vi "平面三体问题v7.vi"() -> ()   [LabVIEW 2018]
uses:
  <vilib>/Analysis/1siggen.llb/Ramp Pattern by Delta.vi
  <vilib>/gmath/NI_Gmath.lvlib
  <vilib>/Analysis/NI_AALBase.lvlib
  <vilib>/ptbypt/NI_PtbyPt.lvlib
panel:
  in  "时间":dbl=10.0 min=0.0
  in  "步长":dbl=0.0005 min=1e-20 format="%0.1e"
  in  "m1":string
  in  "m2":string
  in  "m3":string
  in  "数据计算？":bool
  in  "求解精度":dbl=1e-07 min=1e-20 format="%0.1e"
  out "t":dbl format="%.5f"
  out "d12":dbl format="%.5f"
  out "d23":dbl format="%.5f"
  out "d13":dbl format="%.5f"
  out "s1":dbl format="%.5f"
  out "s2":dbl format="%.5f"
  out "s3":dbl format="%.5f"
  out "p3":string
  out "p1":string
  out "p2 2":string
  out "v1":string
  out "v2":string
  out "v3":string
  out "vmc":string
  out "smc":dbl format="%.5f"
  out "pmc":string
  in  "物体1半径":dbl=1.0 format="%0.2f"
  in  "物体2半径":dbl=1.0 format="%0.2f"
  in  "物体3半径":dbl=1.0 format="%0.2f"
  in  "画圆点数":dbl=256.0 format="%0.2f"
  in  "显示物体半径？":bool
  out "?":T1(graph)
  out "dmax12":dbl format="%.5f"
  out "dmax23":dbl format="%.5f"
  out "dmax13":dbl format="%.5f"
  out "dmin12":dbl format="%.5f"
  out "dmin23":dbl format="%.5f"
  out "dmin13":dbl format="%.5f"
  out "tdmin12":dbl format="%.5f"
  out "tdmax12":dbl format="%.5f"
  out "tdmin23":dbl format="%.5f"
  out "tdmax23":dbl format="%.5f"
  out "tdmax13":dbl format="%.5f"
  out "tdmin13":dbl format="%.5f"
  in  "p2":string
  in  "p3":string
  in  "v1":string
  in  "v2":string
  in  "v3":string
  in  "自动缩放？":bool
  out "smax1":dbl format="%.5g"
  out "smax2":dbl format="%.5g"
  out "smax3":dbl format="%.5g"
  out "smin1":dbl format="%.5g"
  out "smin2":dbl format="%.5g"
  out "smin3":dbl format="%.5g"
  out "tsmax2":dbl format="%.5g"
  out "tsmin2":dbl format="%.5g"
  out "tsmax3":dbl format="%.5g"
  out "tsmin3":dbl format="%.5g"
  out "tsmax1":dbl format="%.5g"
  out "tsmin1":dbl format="%.5g"
  in  "p1":string
  in  "极坐标速度？":bool
  in  "国际单位？":bool
  in  "?":bool
  in  "?":bool
  in  "?":bool
  in  "?":bool
  # "平面三体问题"
  # "三体运动"
  # "参数计算"
  # "显示配置"
  # "高级"
  # "计算配置"
  # "参数输入"
  # "孙家琛\nsjcsjc2001@163.com\n2019.2.19\nSSS"
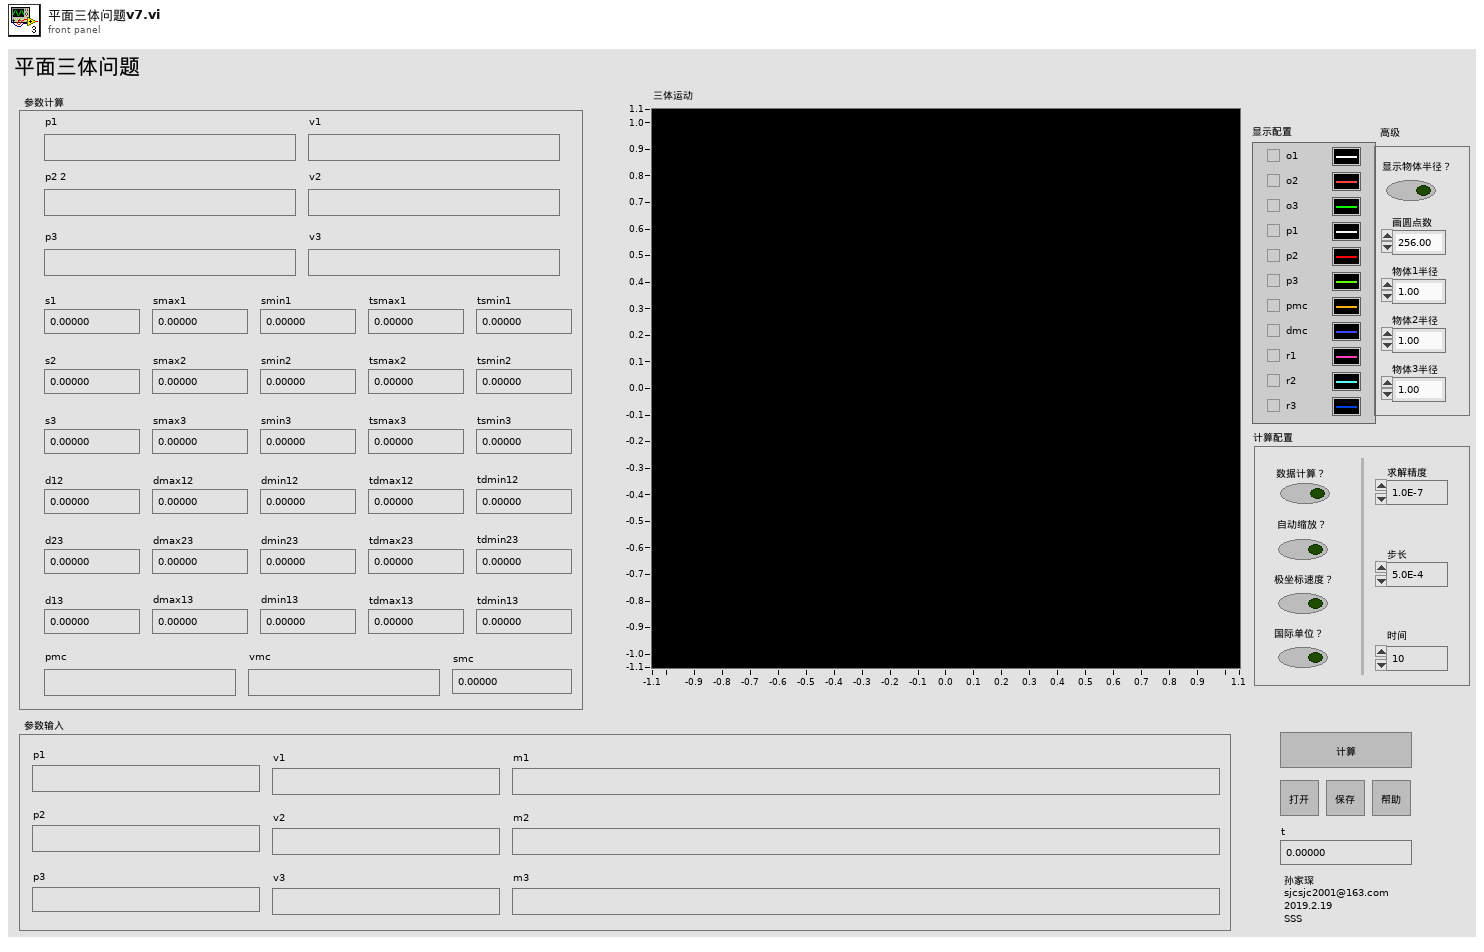
[diagram p1: front panel]
types:
  T1 = cluster{"X Values (solution)":dbl[], "X Values (solution)":dbl[]}[]
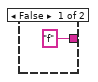
[diagram p4: hidden frame]
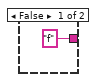
[diagram p5: hidden frame]
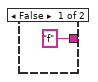
[diagram p6: hidden frame]
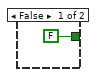
[diagram p8: hidden frame]
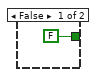
[diagram p9: hidden frame]
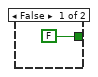
[diagram p10: hidden frame]
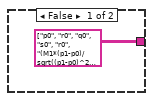
[diagram p11: hidden frame]
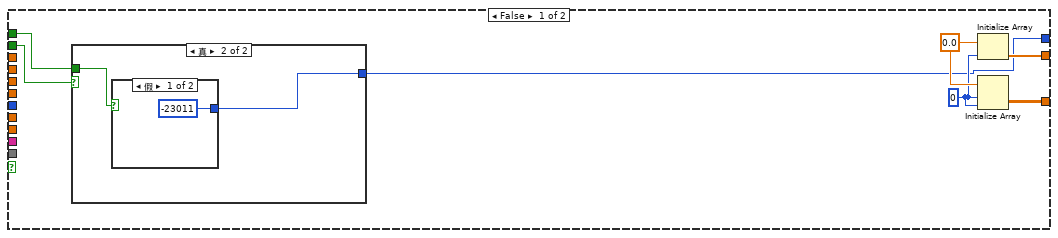
[diagram p13: hidden frame]
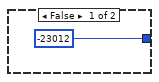
[diagram p14: hidden frame]
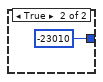
[diagram p15: hidden frame]
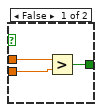
[diagram p16: hidden frame]
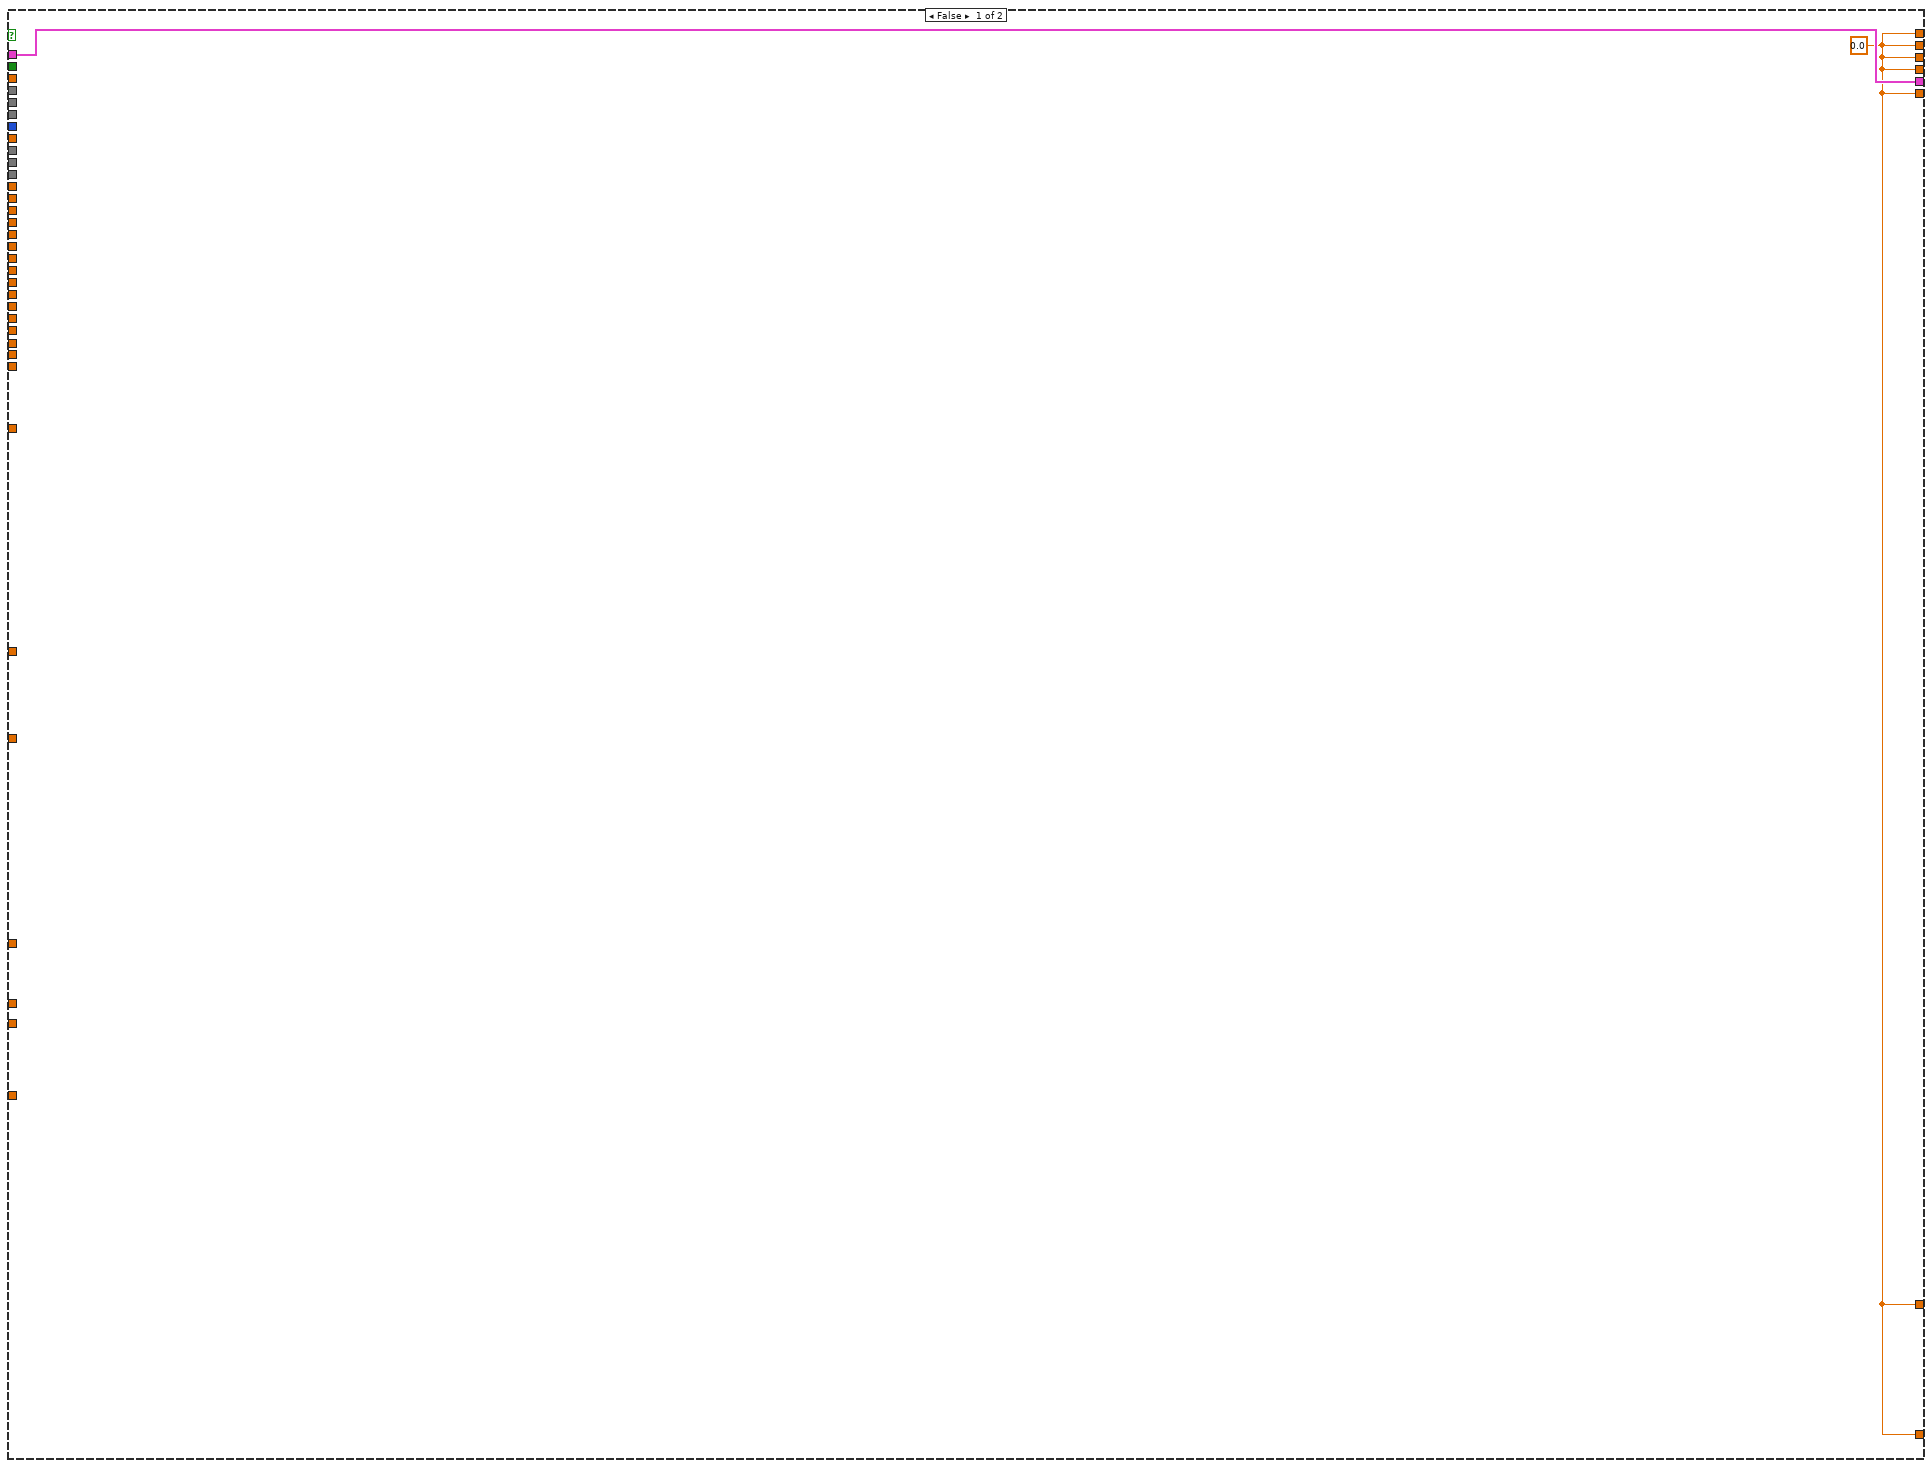
[diagram p19: hidden frame]
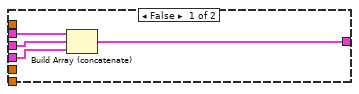
[diagram p20: hidden frame]
diagram:
  n1 = flat-sequence {
    frame #0 {
      n2 = while {
        stop <- "?" stop-if-true
        n3 = case shown="真" "?" {
          frame False {
          }
          frame True {
            n4 = property on="极坐标速度？" class="Bool (严格)"() -> ("Value"=w20:bool)  [unwired: 2 in, 2 out]
            n5 = property on="显示物体半径？" class="Bool (严格)"() -> ("Value"=w14:bool)  [unwired: 2 in, 2 out]
            n6 = property on="国际单位？" class="Bool (严格)"() -> ("Value"=w19:bool)  [unwired: 2 in, 2 out]
            n7 = case shown="真" w20 {
              tunnel: ["f" "p"] -> w18
              frame False {
              }
              frame True {
              }
            }
            n8 = case shown="真" w19 {
              tunnel: ["f" "i"] -> w17
              frame False {
              }
              frame True {
              }
            }
            n9 = case shown="真" w14 {
              tunnel: ["f" "r"] -> w13
              frame False {
              }
              frame True {
              }
            }
            n10 = property on="时间" class="DigNum (严格)"() -> ("Value"=w16:dbl)  [unwired: 2 in, 2 out]
            n11 = property on="1" class="DigNum (严格)"() -> ("Value"=w12:dbl)  [unwired: 2 in, 2 out]
            n12 = property on="2" class="DigNum (严格)"() -> ("Value"=w10:dbl)  [unwired: 2 in, 2 out]
            n13 = property on="3" class="DigNum (严格)"() -> ("Value"=w7:dbl)  [unwired: 2 in, 2 out]
            n14 = Number To Fractional String(number=w16) -> (F-format string=w15:string)  [unwired: 3 in]
            n15 = Number To Fractional String(number=w12) -> (F-format string=w11:string)  [unwired: 3 in]
            n16 = Number To Fractional String(number=w10) -> (F-format string=w9:string)  [unwired: 3 in]
            n17 = Number To Fractional String(number=w7) -> (F-format string=w6:string)  [unwired: 3 in]
            n18 = property on="p1" class="Str"() -> ("Value"=w28:string)  [unwired: 2 in, 2 out]
            n19 = property on="p2" class="Str"() -> ("Value"=w27:string)  [unwired: 2 in, 2 out]
            n20 = property on="p3" class="Str"() -> ("Value"=w26:string)  [unwired: 2 in, 2 out]
            n21 = property on="v1" class="Str"() -> ("Value"=w25:string)  [unwired: 2 in, 2 out]
            n22 = property on="v2" class="Str"() -> ("Value"=w24:string)  [unwired: 2 in, 2 out]
            n23 = property on="v3" class="Str"() -> ("Value"=w23:string)  [unwired: 2 in, 2 out]
            n24 = property on="m1" class="Str"() -> ("Value"=w29:string)  [unwired: 2 in, 2 out]
            n25 = property on="m2" class="Str"() -> ("Value"=w30:string)  [unwired: 2 in, 2 out]
            n26 = property on="m3" class="Str"() -> ("Value"=w21:string)  [unwired: 2 in, 2 out]
            n27 = call <vilib>:"Space Constant.vi"() -> ("String"=w8:string)
            n28 = Concatenate Strings(w28, w8, w27, w8, w26, w8, w25, w8, w24, w8, w23, w8, w29, w8, w30, w8, w21, w8, w18, w8, w17, w8, w15, w8, w13, w8, w11, w8, w9, w8, w6) -> (w22:string)
            n29 = Write to Text File(text=w22) -> ()  [unwired: 3 in, 3 out]
          }
        }
        n30 = case shown="真" "?" {
          frame False {
          }
          frame True {
            n31 = One Button Dialog(message="帮助：\nt：运行时间\nr1：物体1曲线；r2：物体2曲线；r3：物体3曲线\np1：物体1位置；p2：物体2位置；p3：物体3位置\nm1：物体1质量；m2：物体2质量；m3：物体3质量\nv1：物体1速度；v2：物体2速度；v3：物体3速度\ns1：物体1速率；s2：物体2速率；s3：物体3速率\nsmax1：物体1最大速率；smax2：物体2最大速率；smax3：物体3最大速率\nsmin1：物体1最小速率；smin2：物体2最小速率；smin3：物体3最小速率\ntsmax1：物体1最大速率时间；tsmax2：物体2最大速率时间；tsmax3：物体3最大速率时间\ntsmin1：物体1最小速率时间；tsmin2：物体2最小速率时间；tsmin3：物体3最小速率时间\nd12：物体1-物体2距离；d23：物体2-物体3距离；d13：物体1-物体3距离\ndmax12：物体1-物体2最大距离；dmax23：物体2-物体3最大距离；dmax13：物体1-物体3最大距离\ndmin12：物体1-物体2最小距离；dmin23：物体2-物体3最小距离；dmin13：物体1-物体3最小距离\ntdmax12：物体1-物体2最大距离时间；tdmax23：物体2-物体3最大距离时间；tdmax13：物体1-物体3最大距离时间\ntdmin12：物体1-物体2最小距离时间；tdmin23：物体2-物体3最小距离时间；tdmin13：物体1-物体3最小距离时间\npmc：系统质心位置；vmc：系统质心速度；smc：系统质心速率；dmc：系统质心方向\n\n（注：位置和速度使用向量表示，格式为(x,y)）" ("消息")) -> ()  [unwired: 1 in, 1 out]
          }
        }
        n32 = case shown="真" "?" {
          frame False {
          }
          frame True {
            n33 = Read from Text File() -> (text=w81:string)  [unwired: 4 in, 3 out]
            n34 = call <vilib>:"Space Constant.vi"() -> ("String"=w40:string)
            n35 = Search/Split String(string=w81, search string/char (-)=w40) -> (substring before match=w111:string, match + rest of string=w110:string)  [unwired: 1 in, 1 out]
            n36 = property on="p1" class="Str"("Value"=w111) -> ()  [unwired: 2 in, 2 out]
            n37 = String Subset(string=w110, offset (0)=1 ("偏移量(0)")) -> (substring=w108:string)  [unwired: 1 in]
            n38 = Search/Split String(string=w108, search string/char (-)=w40) -> (substring before match=w107:string, match + rest of string=w61:string)  [unwired: 1 in, 1 out]
            n39 = property on="p2" class="Str"("Value"=w107) -> ()  [unwired: 2 in, 2 out]
            n40 = String Subset(string=w61, offset (0)=1 ("偏移量(0)")) -> (substring=w105:string)  [unwired: 1 in]
            n41 = Search/Split String(string=w105, search string/char (-)=w40) -> (substring before match=w104:string, match + rest of string=w101:string)  [unwired: 1 in, 1 out]
            n42 = property on="p3" class="Str"("Value"=w104) -> ()  [unwired: 2 in, 2 out]
            n43 = String Subset(string=w101, offset (0)=1 ("偏移量(0)")) -> (substring=w102:string)  [unwired: 1 in]
            n44 = Search/Split String(string=w102, search string/char (-)=w40) -> (substring before match=w100:string, match + rest of string=w97:string)  [unwired: 1 in, 1 out]
            n45 = property on="v1" class="Str"("Value"=w100) -> ()  [unwired: 2 in, 2 out]
            n46 = String Subset(string=w97, offset (0)=1 ("偏移量(0)")) -> (substring=w98:string)  [unwired: 1 in]
            n47 = Search/Split String(string=w98, search string/char (-)=w40) -> (substring before match=w96:string, match + rest of string=w93:string)  [unwired: 1 in, 1 out]
            n48 = property on="v2" class="Str"("Value"=w96) -> ()  [unwired: 2 in, 2 out]
            n49 = String Subset(string=w93, offset (0)=1 ("偏移量(0)")) -> (substring=w94:string)  [unwired: 1 in]
            n50 = Search/Split String(string=w94, search string/char (-)=w40) -> (substring before match=w92:string, match + rest of string=w89:string)  [unwired: 1 in, 1 out]
            n51 = property on="v3" class="Str"("Value"=w92) -> ()  [unwired: 2 in, 2 out]
            n52 = String Subset(string=w89, offset (0)=1 ("偏移量(0)")) -> (substring=w90:string)  [unwired: 1 in]
            n53 = Search/Split String(string=w90, search string/char (-)=w40) -> (substring before match=w88:string, match + rest of string=w85:string)  [unwired: 1 in, 1 out]
            n54 = property on="m1" class="Str"("Value"=w88) -> ()  [unwired: 2 in, 2 out]
            n55 = String Subset(string=w85, offset (0)=1 ("偏移量(0)")) -> (substring=w86:string)  [unwired: 1 in]
            n56 = Search/Split String(string=w86, search string/char (-)=w40) -> (substring before match=w84:string, match + rest of string=w82:string)  [unwired: 1 in, 1 out]
            n57 = property on="m2" class="Str"("Value"=w84) -> ()  [unwired: 2 in, 2 out]
            n58 = String Subset(string=w82, offset (0)=1 ("偏移量(0)")) -> (substring=w80:string)  [unwired: 1 in]
            n59 = Search/Split String(string=w80, search string/char (-)=w40) -> (substring before match=w79:string, match + rest of string=w71:string)  [unwired: 1 in, 1 out]
            n60 = property on="m3" class="Str"("Value"=w79) -> ()  [unwired: 2 in, 2 out]
            n61 = String Subset(string=w71, offset (0)=1 ("偏移量(0)")) -> (substring=w70:string)  [unwired: 1 in]
            n62 = Search/Split String(string=w70, search string/char (-)=w40) -> (substring before match=w69:string, match + rest of string=w67:string)  [unwired: 1 in, 1 out]
            n63 = String Subset(string=w67, offset (0)=1 ("偏移量(0)")) -> (substring=w66:string)  [unwired: 1 in]
            n64 = Equal?(x=w69, y="p") -> (x = y?=w78:bool)
            n65 = Search/Split String(string=w66, search string/char (-)=w40) -> (substring before match=w65:string, match + rest of string=w63:string)  [unwired: 1 in, 1 out]
            n66 = case shown="真" w78 {
              tunnel: [FALSE TRUE] -> w74
              frame False {
              }
              frame True {
              }
            }
            n67 = Equal?(x=w65, y="i") -> (x = y?=w76:bool)
            n68 = String Subset(string=w63, offset (0)=1 ("偏移量(0)")) -> (substring=w60:string)  [unwired: 1 in]
            n69 = Search/Split String(string=w60, search string/char (-)=w40) -> (substring before match=w59:string, match + rest of string=w58:string)  [unwired: 1 in, 1 out]
            n70 = case shown="真" w76 {
              tunnel: [FALSE TRUE] -> w73
              frame False {
              }
              frame True {
              }
            }
            n71 = property on="极坐标速度？" class="Bool (严格)"("Value"=w74) -> ()  [unwired: 2 in, 2 out]
            n72 = Fract/Exp String To Number(string=w59) -> (number=w62:dbl)  [unwired: 3 in, 1 out]
            n73 = String Subset(string=w58, offset (0)=1 ("偏移量(0)")) -> (substring=w56:string)  [unwired: 1 in]
            n74 = property on="时间" class="DigNum (严格)"("Value"=w62) -> ()  [unwired: 2 in, 2 out]
            n75 = Search/Split String(string=w56, search string/char (-)=w40) -> (substring before match=w54:string, match + rest of string=w51:string)  [unwired: 1 in, 1 out]
            n76 = property on="国际单位？" class="Bool (严格)"("Value"=w73) -> ()  [unwired: 2 in, 2 out]
            n77 = Equal?(x=w54, y="r") -> (x = y?=w53:bool)
            n78 = String Subset(string=w51, offset (0)=1 ("偏移量(0)")) -> (substring=w50:string)  [unwired: 1 in]
            n79 = Search/Split String(string=w50, search string/char (-)=w40) -> (substring before match=w48:string, match + rest of string=w46:string)  [unwired: 1 in, 1 out]
            n80 = case shown="真" w53 {
              tunnel: [FALSE TRUE] -> w37
              frame False {
              }
              frame True {
              }
            }
            n81 = Fract/Exp String To Number(string=w48) -> (number=w49:dbl)  [unwired: 3 in, 1 out]
            n82 = String Subset(string=w46, offset (0)=1 ("偏移量(0)")) -> (substring=w45:string)  [unwired: 1 in]
            n83 = property on="1" class="DigNum (严格)"("Value"=w49) -> ()  [unwired: 2 in, 2 out]
            n84 = Search/Split String(string=w45, search string/char (-)=w40) -> (substring before match=w43:string, match + rest of string=w41:string)  [unwired: 1 in, 1 out]
            n85 = property on="显示物体半径？" class="Bool (严格)"("Value"=w37) -> ()  [unwired: 2 in, 2 out]
            n86 = Fract/Exp String To Number(string=w43) -> (number=w44:dbl)  [unwired: 3 in, 1 out]
            n87 = String Subset(string=w41, offset (0)=1 ("偏移量(0)")) -> (substring=w39:string)  [unwired: 1 in]
            n88 = property on="2" class="DigNum (严格)"("Value"=w44) -> ()  [unwired: 2 in, 2 out]
            n89 = Fract/Exp String To Number(string=w39) -> (number=w38:dbl)  [unwired: 3 in, 1 out]
            n90 = property on="3" class="DigNum (严格)"("Value"=w38) -> ()  [unwired: 2 in, 2 out]
          }
        }
      }
    }
    frame #1 {
      w125 = 1.0 ("cycles")
      w124 = 90.0 ("phase(degrees)")
      w181 = "t" ("time")
      n91 = Search/Split String(string="v1", search string/char (-)="," ("搜索字符串/字符(-)")) -> (substring before match=w313:string, offset of match=w298:i32)  [unwired: 1 in, 1 out]
      n92 = Search/Split String(string="v2", search string/char (-)="," ("搜索字符串/字符(-)")) -> (substring before match=w296:string, offset of match=w281:i32)  [unwired: 1 in, 1 out]
      n93 = Search/Split String(string="v3", search string/char (-)="," ("搜索字符串/字符(-)")) -> (substring before match=w279:string, offset of match=w264:i32)  [unwired: 1 in, 1 out]
      n94 = Search/Split String(string="v1", search string/char (-)="(" ("搜索字符串/字符(-)")) -> (offset of match=w309:i32)  [unwired: 1 in, 2 out]
      n95 = Search/Split String(string="v1", search string/char (-)=")" ("搜索字符串/字符(-)")) -> (offset of match=w310:i32)  [unwired: 1 in, 2 out]
      n96 = Search/Split String(string="v2", search string/char (-)="(" ("搜索字符串/字符(-)")) -> (offset of match=w292:i32)  [unwired: 1 in, 2 out]
      n97 = Search/Split String(string="v2", search string/char (-)=")" ("搜索字符串/字符(-)")) -> (offset of match=w293:i32)  [unwired: 1 in, 2 out]
      n98 = Search/Split String(string="v3", search string/char (-)="(" ("搜索字符串/字符(-)")) -> (offset of match=w275:i32)  [unwired: 1 in, 2 out]
      n99 = Search/Split String(string="v3", search string/char (-)=")" ("搜索字符串/字符(-)")) -> (offset of match=w276:i32)  [unwired: 1 in, 2 out]
      n100 = Subtract(x=w298, y=w309) -> (x-y=w308:i32)
      n101 = Subtract(x=w310, y=w298) -> (x-y=w299:i32)
      n102 = Subtract(x=w281, y=w292) -> (x-y=w291:i32)
      n103 = Subtract(x=w293, y=w281) -> (x-y=w282:i32)
      n104 = Subtract(x=w264, y=w275) -> (x-y=w274:i32)
      n105 = Subtract(x=w276, y=w264) -> (x-y=w265:i32)
      n106 = Add(x=w309, y=1) -> (x+y=w305:i32)
      n107 = Add(x=w298, y=1) -> (x+y=w301:i32)
      n108 = Add(x=w292, y=1) -> (x+y=w288:i32)
      n109 = Add(x=w281, y=1) -> (x+y=w284:i32)
      n110 = Add(x=w275, y=1) -> (x+y=w271:i32)
      n111 = Add(x=w264, y=1) -> (x+y=w267:i32)
      n112 = Subtract(x=w308, y=1) -> (x-y=w304:i32)
      n113 = Subtract(x=w299, y=1) -> (x-y=w300:i32)
      n114 = Subtract(x=w291, y=1) -> (x-y=w287:i32)
      n115 = Subtract(x=w282, y=1) -> (x-y=w283:i32)
      n116 = Subtract(x=w274, y=1) -> (x-y=w270:i32)
      n117 = Subtract(x=w265, y=1) -> (x-y=w266:i32)
      n118 = String Subset(string=w313, offset (0)=w305, length (rest)=w304) -> (substring=w162:string)
      n119 = String Subset(string="v1", offset (0)=w301, length (rest)=w300) -> (substring=w168:string)
      n120 = String Subset(string=w296, offset (0)=w288, length (rest)=w287) -> (substring=w166:string)
      n121 = String Subset(string="v2", offset (0)=w284, length (rest)=w283) -> (substring=w165:string)
      n122 = String Subset(string=w279, offset (0)=w271, length (rest)=w270) -> (substring=w163:string)
      n123 = String Subset(string="v3", offset (0)=w267, length (rest)=w266) -> (substring=w164:string)
      n124 = case shown="真" "极坐标速度？" {
        tunnel: w168 -> [w409 w421]
        tunnel: w166 -> [w413 w441]
        tunnel: w165 -> [w412 w440]
        tunnel: w164 -> [w410 w439]
        tunnel: w163 -> [w411 w438]
        tunnel: w162 -> [w414 w437]
        tunnel: [w414 w431] -> w161
        tunnel: [w409 w430] -> w160
        tunnel: [w413 w427] -> w159
        tunnel: [w412 w426] -> w158
        tunnel: [w411 w423] -> w157
        tunnel: [w410 w422] -> w156
        frame False {
        }
        frame True {
          n125 = Fract/Exp String To Number(string=w437) -> (number=w436:dbl)  [unwired: 3 in, 1 out]
          n126 = Fract/Exp String To Number(string=w421) -> (number=w419:dbl)  [unwired: 3 in, 1 out]
          n127 = Fract/Exp String To Number(string=w441) -> (number=w435:dbl)  [unwired: 3 in, 1 out]
          n128 = Fract/Exp String To Number(string=w440) -> (number=w417:dbl)  [unwired: 3 in, 1 out]
          n129 = Fract/Exp String To Number(string=w438) -> (number=w434:dbl)  [unwired: 3 in, 1 out]
          n130 = Fract/Exp String To Number(string=w439) -> (number=w415:dbl)  [unwired: 3 in, 1 out]
          n131 = expression code="(x/180.0)*pi" "角度转换至弧度"(w419) -> (w420:dbl)
          n132 = expression code="(x/180.0)*pi" "角度转换至弧度"(w417) -> (w418:dbl)
          n133 = expression code="(x/180.0)*pi" "角度转换至弧度"(w415) -> (w416:dbl)
          n134 = call <vilib>:"1D Polar to Rectangular PtByPt.vi"("phase"=w420, "magnitude"=w436) -> ("y"=w432:dbl, "x"=w433:dbl)
          n135 = call <vilib>:"1D Polar to Rectangular PtByPt.vi"("phase"=w418, "magnitude"=w435) -> ("y"=w428:dbl, "x"=w429:dbl)
          n136 = call <vilib>:"1D Polar to Rectangular PtByPt.vi"("phase"=w416, "magnitude"=w434) -> ("y"=w424:dbl, "x"=w425:dbl)
          n137 = Number To Fractional String(number=w433) -> (F-format string=w431:string)  [unwired: 3 in]
          n138 = Number To Fractional String(number=w432) -> (F-format string=w430:string)  [unwired: 3 in]
          n139 = Number To Fractional String(number=w429) -> (F-format string=w427:string)  [unwired: 3 in]
          n140 = Number To Fractional String(number=w428) -> (F-format string=w426:string)  [unwired: 3 in]
          n141 = Number To Fractional String(number=w425) -> (F-format string=w423:string)  [unwired: 3 in]
          n142 = Number To Fractional String(number=w424) -> (F-format string=w422:string)  [unwired: 3 in]
        }
      }
      n143 = case shown="真" "国际单位？" {
        tunnel: [string[][] [["p0", "r0"], ["q0", "s0"], ["r0", "(M1*(p1-p0)/sqrt((p1-p0)^2+(q1-q0)^2)^3+M2*(p2-p0)/sqrt((p2-p0)^2+(q2-q0)^2)^3)"], ["s0", "(M1*(q1-q0)/sqrt((p1-p0)^2+(q1-q0)^2)^3+M2*(q2-q0)/sqrt((p2-p0)^2+(q2-q0)^2)^3)"], ["p1", "r1"], ["q1", "s1"], ["r1", "(M2*(p2-p1)/sqrt((p2-p1)^2+(q2-q1)^2)^3+M0*(p0-p1)/sqrt((p0-p1)^2+(q0-q1)^2)^3)"], ["s1", "(M2*(q2-q1)/sqrt((p2-p1)^2+(q2-q1)^2)^3+M0*(q0-q1)/sqrt((p0-p1)^2+(q0-q1)^2)^3)"], ["p2", "r2"], ["q2", "s2"], ["r2", "(M0*(p0-p2)/sqrt((p0-p2)^2+(q0-q2)^2)^3+M1*(p1-p2)/sqrt((p1-p2)^2+(q1-q2)^2)^3)"], ["s2", "(M0*(q0-q2)/sqrt((p0-p2)^2+(q0-q2)^2)^3+M1*(q1-q2)/sqrt((p1-p2)^2+(q1-q2)^2)^3)"]] ("公式表格") string[][] [["p0", "r0"], ["q0", "s0"], ["r0", "(M1*(p1-p0)/sqrt((p1-p0)^2+(q1-q0)^2)^3+M2*(p2-p0)/sqrt((p2-p0)^2+(q2-q0)^2)^3)*0.00000000006674"], ["s0", "(M1*(q1-q0)/sqrt((p1-p0)^2+(q1-q0)^2)^3+M2*(q2-q0)/sqrt((p2-p0)^2+(q2-q0)^2)^3)*0.00000000006674"], ["p1", "r1"], ["q1", "s1"], ["r1", "(M2*(p2-p1)/sqrt((p2-p1)^2+(q2-q1)^2)^3+M0*(p0-p1)/sqrt((p0-p1)^2+(q0-q1)^2)^3)*0.00000000006674"], ["s1", "(M2*(q2-q1)/sqrt((p2-p1)^2+(q2-q1)^2)^3+M0*(q0-q1)/sqrt((p0-p1)^2+(q0-q1)^2)^3)*0.00000000006674"], ["p2", "r2"], ["q2", "s2"], ["r2", "(M0*(p0-p2)/sqrt((p0-p2)^2+(q0-q2)^2)^3+M1*(p1-p2)/sqrt((p1-p2)^2+(q1-q2)^2)^3)*0.00000000006674"], ["s2", "(M0*(q0-q2)/sqrt((p0-p2)^2+(q0-q2)^2)^3+M1*(q1-q2)/sqrt((p1-p2)^2+(q1-q2)^2)^3)*0.00000000006674"]] ("公式表格")] -> w149
        frame False {
        }
        frame True {
        }
      }
      n144 = Fract/Exp String To Number(string="m1") -> (number=w172:dbl)  [unwired: 3 in, 1 out]
      n145 = Fract/Exp String To Number(string="m2") -> (number=w171:dbl)  [unwired: 3 in, 1 out]
      n146 = Fract/Exp String To Number(string="m3") -> (number=w170:dbl)  [unwired: 3 in, 1 out]
      n147 = Number To Fractional String(number=w172) -> (F-format string=w222:string)  [unwired: 3 in]
      n148 = Number To Fractional String(number=w171) -> (F-format string=w221:string)  [unwired: 3 in]
      n149 = Number To Fractional String(number=w170) -> (F-format string=w220:string)  [unwired: 3 in]
      n150 = Bundle("M0", w222) -> (w400:cluster{string, string})  [unwired: 1 out]
      n151 = Bundle("M1", w221) -> (w399:cluster{string, string})  [unwired: 1 out]
      n152 = Bundle("M2", w220) -> (w398:cluster{string, string})  [unwired: 1 out]
      n153 = Search/Split String(string="p1", search string/char (-)="(" ("搜索字符串/字符(-)")) -> (offset of match=w364:i32)  [unwired: 1 in, 2 out]
      n154 = Search/Split String(string="p2", search string/char (-)="(" ("搜索字符串/字符(-)")) -> (offset of match=w346:i32)  [unwired: 1 in, 2 out]
      n155 = Search/Split String(string="p3", search string/char (-)="(" ("搜索字符串/字符(-)")) -> (offset of match=w328:i32)  [unwired: 1 in, 2 out]
      n156 = Search/Split String(string="p1", search string/char (-)=")" ("搜索字符串/字符(-)")) -> (substring before match=w150:string, offset of match=w365:i32)  [unwired: 1 in, 1 out]
      n157 = Search/Split String(string="p2", search string/char (-)=")" ("搜索字符串/字符(-)")) -> (substring before match=w153:string, offset of match=w347:i32)  [unwired: 1 in, 1 out]
      n158 = Search/Split String(string="p3", search string/char (-)=")" ("搜索字符串/字符(-)")) -> (substring before match=w151:string, offset of match=w329:i32)  [unwired: 1 in, 1 out]
      n159 = Search/Split String(string="p1", search string/char (-)="," ("搜索字符串/字符(-)")) -> (substring before match=w368:string, offset of match=w353:i32)  [unwired: 1 in, 1 out]
      n160 = Search/Split String(string="p2", search string/char (-)="," ("搜索字符串/字符(-)")) -> (substring before match=w350:string, offset of match=w335:i32)  [unwired: 1 in, 1 out]
      n161 = Search/Split String(string="p3", search string/char (-)="," ("搜索字符串/字符(-)")) -> (substring before match=w332:string, offset of match=w317:i32)  [unwired: 1 in, 1 out]
      n162 = Subtract(x=w353, y=w364) -> (x-y=w363:i32)
      n163 = Subtract(x=w365, y=w353) -> (x-y=w354:i32)
      n164 = Subtract(x=w335, y=w346) -> (x-y=w345:i32)
      n165 = Subtract(x=w347, y=w335) -> (x-y=w336:i32)
      n166 = Subtract(x=w317, y=w328) -> (x-y=w327:i32)
      n167 = Subtract(x=w329, y=w317) -> (x-y=w318:i32)
      n168 = Add(x=w346, y=1) -> (x+y=w342:i32)
      n169 = Add(x=w335, y=1) -> (x+y=w338:i32)
      n170 = Add(x=w328, y=1) -> (x+y=w324:i32)
      n171 = Add(x=w317, y=1) -> (x+y=w320:i32)
      n172 = Build Array(w400, w399, w398) -> (w397:cluster{string, string}[])
      n173 = Add(x=w364, y=1) -> (x+y=w360:i32)
      n174 = Subtract(x=w363, y=1) -> (x-y=w359:i32)
      n175 = Add(x=w353, y=1) -> (x+y=w356:i32)
      n176 = Subtract(x=w354, y=1) -> (x-y=w355:i32)
      n177 = Subtract(x=w345, y=1) -> (x-y=w341:i32)
      n178 = Subtract(x=w336, y=1) -> (x-y=w337:i32)
      n179 = Subtract(x=w327, y=1) -> (x-y=w323:i32)
      n180 = Subtract(x=w318, y=1) -> (x-y=w319:i32)
      n181 = Index Array(array=w149, index (col) #1=0 ("disabled index (col)"), index (col) #2=1 ("index (col)")) -> (element #1=w176:string[], element #2=w386:string[])  [unwired: 2 in]
      n182 = for {
        tunnel: w386 -> [w874] mode=indexing
        tunnel: w397 -> [w872]
        tunnel: [w873] -> w175 mode=indexing
        n183 = call <vilib>:"Substitute Variables.vi"("Substitution Rules"=w872, "original formula"=w874) -> ("formula after substitution"=w873:string)  [unwired: 1 in, 1 out]
      }
      n184 = String Subset(string=w368, offset (0)=w360, length (rest)=w359) -> (substring=w154:string)
      n185 = String Subset(string=w150, offset (0)=w356, length (rest)=w355) -> (substring=w352:string)
      n186 = String Subset(string=w350, offset (0)=w342, length (rest)=w341) -> (substring=w167:string)
      n187 = String Subset(string=w153, offset (0)=w338, length (rest)=w337) -> (substring=w334:string)
      n188 = String Subset(string=w332, offset (0)=w324, length (rest)=w323) -> (substring=w316:string)
      n189 = String Subset(string=w151, offset (0)=w320, length (rest)=w319) -> (substring=w315:string)
      n190 = Build Array(w154, w352, w161, w160, w167, w334, w159, w158, w316, w315, w157, w156) -> (w383:string[])
      n191 = Fract/Exp String To Number(string=w383) -> (number=w180:dbl[])  [unwired: 3 in, 1 out]
      n192 = call <vilib>:"Cash Karp Check.vi"("F(X,t)"=w175, "X"=w176, "time"=w181, "X(0)"=w180) -> ("system OK"=w187:bool, "zero array"=w182:dbl[], "result"=w184:dbl[][], "table"=w183:i32[][][])  [unwired: 1 in, 3 out]
      n193 = Greater Than 0?(x="求解精度") -> (x > 0?=w186:bool)
      n194 = Greater Than 0?(x="步长") -> (x > 0?=w185:bool)
      n195 = Compound Arithmetic op=AND(w186, w185, w187) -> (w188:bool)
      n196 = case shown="真" w188 {
        tunnel: w180 -> [_ w473]
        tunnel: [w445 w468] -> w174
        tunnel: [w446 w467] -> w173
        tunnel: "步长" -> [_ w463]
        tunnel: "求解精度" -> [_ w465]
        tunnel: [w442 0] -> _
        tunnel: w186 -> [w444 _]
        tunnel: w185 -> [w443 _]
        tunnel: w184 -> [_ w456]
        tunnel: w183 -> [_ w457]
        tunnel: w182 -> [_ w460]
        tunnel: w176 -> [_ w458]
        tunnel: w181 -> [_ w459]
        tunnel: "时间" -> [_ w455]
        frame False {
          w447 = 0
          w448 = 0.0
          n197 = case shown="真" w444 {
            tunnel: w443 -> [_ w451]
            tunnel: [-23012 w450] -> w442
            frame False {
            }
            frame True {
              n198 = case shown="假" w451 {
                tunnel: [-23011 -23010] -> w450
                frame False {
                }
                frame True {
                }
              }
            }
          }
          n199 = Initialize Array(w448, w447) -> (w445:dbl[])
          n200 = Initialize Array(w448, w447, w447) -> (w446:dbl[][])
        }
        frame True {
          w454 = 0.0 ("time start")
          w466 = 0
          n201 = Greater Or Equal?(x=w454, y=w455) -> (x >= y?=w461:bool)
          n202 = case shown="真" w461 {
            tunnel: w463 -> [w516 w518]
            tunnel: [w516 w517] -> w462
            frame False {
            }
            frame True {
              n203 = Negate(x=w518) -> (-x=w517:dbl)
            }
          }
          n204 = Initialize Array(0.0, 0) -> (w469:dbl[])
          n205 = Initialize Array(0.0, w466, w466) -> (w472:dbl[][])
          n206 = while {
            tunnel: w461 -> [w487]
            shift-left: w472 -> [w501]
            shift-right: [w498] -> w467
            shift-left: w469 -> [w502]
            shift-right: [w499] -> _
            shift-left: w469 -> [w503]
            shift-right: [w500] -> w468
            tunnel: w465 -> [w506]
            shift-left: w462 -> [w497]
            shift-right: [w486] -> _
            tunnel: w455 -> [w475]
            shift-left: w473 -> [w492]
            shift-right: [w493] -> _
            shift-left: w454 -> [w476]
            shift-right: [w485] -> _
            tunnel: w460 -> [w483]
            tunnel: w459 -> [w482]
            tunnel: w458 -> [w481]
            tunnel: w457 -> [w480]
            tunnel: w456 -> [w479]
            tunnel: w457 -> [w478]
            tunnel: w456 -> [w477]
            stop <- w496 continue-if-true
            n207 = Build Array (concatenate)(w503, w476) -> (w500:dbl[])
            n208 = Build Array (concatenate)(w502, w497) -> (w499:dbl[])
            n209 = Build Array (concatenate)(w501, w492) -> (w498:dbl[][])
            n210 = case shown="真" w487 {
              tunnel: w476 -> [w512 w515]
              tunnel: [w511 w514] -> w507
              tunnel: w475 -> [w510 w513]
              frame False {
                n211 = Greater?(x=w512, y=w510) -> (0:w511:bool)
              }
              frame True {
                n212 = Less?(x=w515, y=w513) -> (x < y?=w514:bool)
              }
            }
            n213 = call <vilib>:"Cash Karp General.vi"("X"=w481, "result"=w479, "time"=w482, "table"=w480, "zero"=w483, "yn"=w492, "xn"=w476, "h"=w497) -> ("yn2"=w509:dbl[], "yn1"=w508:dbl[])  [unwired: 2 in]
            n214 = Subtract(x=w508, y=w509) -> (x-y=w491:dbl[])
            n215 = Multiply(x=w491, y=w491) -> (x*y=w490:dbl[])
            n216 = Not(x=w507) -> (.not. x?=w496:bool)
            n217 = Add Array Elements(numeric array=w490) -> (sum=w488:dbl)
            n218 = Square Root(x=w488) -> (sqrt(x)=w489:dbl)
            n219 = Add(x=w489, y=1e-12) -> (x+y=w494:dbl)
            n220 = Divide(x=w506, y=w494) -> (x/y=w505:dbl)
            n221 = Power Of X(1:w505, 2:0.2) -> (0:w484:dbl)
            n222 = Multiply(x=w484, y=w497) -> (x*y=w486:dbl)
            n223 = Add(x=w476, y=w486) -> (x+y=w485:dbl)
            n224 = call <vilib>:"Cash Karp General.vi"("X"=w481, "result"=w477, "time"=w482, "table"=w478, "zero"=w483, "yn"=w492, "xn"=w476, "h"=w486) -> ("yn2"=w493:dbl[])  [unwired: 2 in, 1 out]
          }
        }
      }
      n225 = Transpose 2D Array(2D array=w173) -> (transposed array=w388:dbl[][])
      n226 = call-poly <vilib>:"Ramp Pattern.vi"("end"="时间", "delta"="步长") -> ("Ramp Pattern"=w384:dbl[])  [unwired: 7 in, 2 out]
      n227 = for {
        tunnel: w388 -> [w827] mode=indexing
        tunnel: [w824] -> w395 mode=indexing
        tunnel: w174 -> [w826]
        tunnel: w384 -> [w825]
        w823 = 2 items=["最近", "线性", "样条", "cubic Hermite", "拉格朗日"] ("method")
        n228 = call <vilib>:"in_1d interp prepare arrays.vi"("xi"=w825, "Y"=w827, "X"=w826) -> ("error"=w828:i32, "xi-out"=w830:dbl[], "Y-out"=w831:dbl[], "X-out"=w832:dbl[], "ntimes remaining"=w829:i32)  [unwired: 4 in]
        n229 = case shown="0" w828 {
          selector: w828 -> [_ w871]
          tunnel: w832 -> [w839 _]
          tunnel: w831 -> [w838 _]
          tunnel: w830 -> [w837 _]
          tunnel: w829 -> [w836 _]
          tunnel: [0 ("error") w871] -> _
          tunnel: [w834 _] -> w824
          tunnel: w823 -> [w833 _]
          frame 0 {
            n230 = case shown="1, 默认" w836 {
              selector: w836 -> [_ w845]
              tunnel: w839 -> [w844 w850]
              tunnel: w838 -> [w843 w847]
              tunnel: w837 -> [w840 _]
              tunnel: [w842 w848] -> w834
              tunnel: w833 -> [w841 w849]
              tunnel: [w840 w846] -> _
              frame 0 {
                n231 = call <vilib>:"in_1d interp.vi"("method"=w841, "xi"=w840, "Y"=w843, "X"=w844) -> ("yi"=w842:dbl[])  [unwired: 6 in, 1 out]
              }
              frame 1, Default {
                n232 = for {
                  N: w845 -> [_]
                  tunnel: w849 -> [w865]
                  shift-right: [w859] -> w846
                  shift-left: w850 -> [w856]
                  shift-right: [w857] -> w848
                  shift-left: w847 -> [w851]
                  n233 = Reverse 1D Array(array=w856) -> (reversed array=w855:dbl[])
                  n234 = Array Size(array=w856) -> (size(s)=w862:i32)
                  n235 = Reverse 1D Array(array=w851) -> (reversed array=w853:dbl[])
                  n236 = Decrement(x=w862) -> (x-1=w861:i32)
                  n237 = Index Array(array=w855) -> (element=w854:dbl)  [unwired: 1 in]
                  n238 = Index Array(array=w853) -> (element=w852:dbl)  [unwired: 1 in]
                  n239 = for {
                    N: w861 -> [_]
                    tunnel: [w870] -> w860 mode=indexing
                    tunnel: w856 -> [w866]
                    i -> [w868]
                    n240 = Add(x=0.5, y=w868) -> (x+y=w867:dbl)
                    n241 = Interpolate 1D Array(1:w867, 2:w866) -> (0:w870:dbl)
                  }
                  n242 = Interleave 1D Arrays(w856, w860) -> (w863:dbl[])
                  n243 = call <vilib>:"in_1d interp.vi"("method"=w865, "xi"=w860, "Y"=w851, "X"=w856) -> ("yi"=w864:dbl[])  [unwired: 6 in, 1 out]
                  n244 = Build Array (concatenate)(w863, w854) -> (w859:dbl[])
                  n245 = Interleave 1D Arrays(w851, w864) -> (w858:dbl[])
                  n246 = Build Array (concatenate)(w858, w852) -> (w857:dbl[])
                }
              }
            }
          }
          frame Default {
          }
        }
      }
      n247 = Index Array(array=w395, index (row) #1=0 ("disabled index (col)"), index (row) #2=1 ("index (col)"), index (row) #3=4 ("index (col)"), index (row) #4=5 ("index (col)"), index (row) #5=8 ("index (col)"), index (row) #6=9 ("index (col)")) -> (element #1=w381:dbl[], element #2=w378:dbl[], element #3=w380:dbl[], element #4=w377:dbl[], element #5=w379:dbl[], element #6=w376:dbl[])  [unwired: 6 in]
      n248 = Array Max & Min(array=w381) -> (max value=w258:dbl, min value=w257:dbl)  [unwired: 2 out]
      n249 = Array Max & Min(array=w380) -> (max value=w256:dbl, min value=w255:dbl)  [unwired: 2 out]
      n250 = Array Max & Min(array=w379) -> (max value=w254:dbl, min value=w253:dbl)  [unwired: 2 out]
      n251 = Array Max & Min(array=w378) -> (max value=w252:dbl, min value=w251:dbl)  [unwired: 2 out]
      n252 = Array Max & Min(array=w377) -> (max value=w250:dbl, min value=w249:dbl)  [unwired: 2 out]
      n253 = Array Max & Min(array=w376) -> (max value=w248:dbl, min value=w247:dbl)  [unwired: 2 out]
      n254 = Bundle("Y-out"=w381, "Y-out"=w378) -> (w406:cluster{"Y-out":dbl[], "Y-out":dbl[]})  [unwired: 1 out]
      n255 = Bundle("Y-out"=w380, "Y-out"=w377) -> (w405:cluster{"Y-out":dbl[], "Y-out":dbl[]})  [unwired: 1 out]
      n256 = Bundle("Y-out"=w379, "Y-out"=w376) -> (w404:cluster{"Y-out":dbl[], "Y-out":dbl[]})  [unwired: 1 out]
      n257 = Build Array(w258, w257, w256, w255, w254, w253) -> (w246:dbl[])
      n258 = Build Array(w252, w251, w250, w249, w248, w247) -> (w245:dbl[])
      n259 = Build Array(w406, w405, w404) -> (w396:cluster{"Y-out":dbl[], "Y-out":dbl[]}[])
      n260 = Array Max & Min(array=w246) -> (max value=w144:dbl, min value=w143:dbl)  [unwired: 2 out]
      n261 = Array Max & Min(array=w245) -> (max value=w140:dbl, min value=w139:dbl)  [unwired: 2 out]
      n262 = Add(x=w144, y=w143) -> (x+y=w141:dbl)
      n263 = Subtract(x=w144, y=w143) -> (x-y=w244:dbl)
      n264 = Subtract(x=w140, y=w139) -> (x-y=w243:dbl)
      n265 = Add(x=w140, y=w139) -> (x+y=w137:dbl)
      n266 = Build Array(w244, w243) -> (w242:dbl[])
      n267 = call <vilib>:"Sine Pattern.vi"("cycles"=w125, "phase(degrees)"=w124, "amplitude"="物体1半径", "samples"="画圆点数") -> ("Sinusoidal Pattern"=w122:dbl[])  [unwired: 1 out]
      n268 = call <vilib>:"Sine Pattern.vi"("cycles"=w125, "amplitude"="物体1半径", "samples"="画圆点数") -> ("Sinusoidal Pattern"=w123:dbl[])  [unwired: 1 in, 1 out]
      n269 = call <vilib>:"Sine Pattern.vi"("cycles"=w125, "amplitude"="物体2半径", "samples"="画圆点数") -> ("Sinusoidal Pattern"=w121:dbl[])  [unwired: 1 in, 1 out]
      n270 = call <vilib>:"Sine Pattern.vi"("cycles"=w125, "phase(degrees)"=w124, "amplitude"="物体2半径", "samples"="画圆点数") -> ("Sinusoidal Pattern"=w120:dbl[])  [unwired: 1 out]
      n271 = Array Max & Min(array=w242) -> (max value=w145:dbl)  [unwired: 3 out]
      n272 = call <vilib>:"Sine Pattern.vi"("cycles"=w125, "phase(degrees)"=w124, "amplitude"="物体3半径", "samples"="画圆点数") -> ("Sinusoidal Pattern"=w118:dbl[])  [unwired: 1 out]
      n273 = call <vilib>:"Sine Pattern.vi"("cycles"=w125, "amplitude"="物体3半径", "samples"="画圆点数") -> ("Sinusoidal Pattern"=w119:dbl[])  [unwired: 1 in, 1 out]
      n274 = for {
        tunnel: w381 -> [w538] mode=indexing
        tunnel: w378 -> [w539] mode=indexing
        tunnel: w380 -> [w537] mode=indexing
        tunnel: w377 -> [w536] mode=indexing
        tunnel: w379 -> [w535] mode=indexing
        tunnel: w376 -> [w534] mode=indexing
        tunnel: w396 -> [w540]
        tunnel: w384 -> [w560] mode=indexing
        tunnel: "数据计算？" -> [w573]
        tunnel: [w563] -> w241 mode=indexing
        tunnel: [w562] -> w236 mode=indexing
        tunnel: [w561] -> w231 mode=indexing
        tunnel: w381 -> [w559]
        tunnel: "步长" -> [w557]
        tunnel: [w556] -> w202
        tunnel: w378 -> [w555]
        tunnel: w380 -> [w554]
        tunnel: w377 -> [w553]
        tunnel: w379 -> [w552]
        tunnel: w376 -> [w551]
        tunnel: w172 -> [w550]
        tunnel: w171 -> [w549]
        tunnel: w170 -> [w548]
        tunnel: w145 -> [w546]
        tunnel: [w545] -> w198 mode=indexing
        tunnel: [w544] -> w190 mode=indexing
        tunnel: [w543] -> w194 mode=indexing
        tunnel: "极坐标速度？" -> [w542]
        tunnel: w123 -> [w533]
        tunnel: w122 -> [w532]
        tunnel: w121 -> [w531]
        tunnel: w120 -> [w530]
        tunnel: w119 -> [w529]
        tunnel: w118 -> [w528]
        i -> [w558]
        n275 = Build Array(w538) -> (w572:dbl[])
        n276 = Build Array(w539) -> (w571:dbl[])
        n277 = Build Array(w537) -> (w569:dbl[])
        n278 = Build Array(w536) -> (w570:dbl[])
        n279 = Build Array(w535) -> (w568:dbl[])
        n280 = Build Array(w534) -> (w567:dbl[])
        n281 = Bundle(w572, w571) -> (w566:cluster{dbl[], dbl[]})  [unwired: 1 out]
        n282 = Bundle(w569, w570) -> (w565:cluster{dbl[], dbl[]})  [unwired: 1 out]
        n283 = Bundle(w568, w567) -> (w564:cluster{dbl[], dbl[]})  [unwired: 1 out]
        n284 = Build Array (concatenate)(w540, w566, w565, w564) -> (w547:cluster{"Y-out":dbl[], "Y-out":dbl[]}[])
        n285 = case shown="真" w573 {
          tunnel: w538 -> [_ w639]
          tunnel: w539 -> [_ w636]
          tunnel: w537 -> [_ w638]
          tunnel: w536 -> [_ w634]
          tunnel: w535 -> [_ w637]
          tunnel: w534 -> [_ w633]
          tunnel: [w574 w757] -> w563
          tunnel: [w574 w756] -> w562
          tunnel: [w574 w755] -> w561
          tunnel: w559 -> [_ w752]
          tunnel: w558 -> [_ w712]
          tunnel: w557 -> [_ w748]
          tunnel: [w574 w709] -> w556
          tunnel: w555 -> [_ w742]
          tunnel: w554 -> [_ w725]
          tunnel: w553 -> [_ w724]
          tunnel: w552 -> [_ w711]
          tunnel: w551 -> [_ w710]
          tunnel: w550 -> [_ w640]
          tunnel: w549 -> [_ w641]
          tunnel: w548 -> [_ w635]
          tunnel: w547 -> [w575 w593]
          tunnel: [w575 w625] -> w541
          tunnel: w546 -> [_ w620]
          tunnel: [w574 w610] -> w545
          tunnel: [w574 w609] -> w544
          tunnel: [w574 w608] -> w543
          tunnel: w542 -> [_ w607]
          tunnel: w539 -> [_ _]
          tunnel: w538 -> [_ _]
          tunnel: w539 -> [_ w588]
          tunnel: w538 -> [_ w587]
          tunnel: w537 -> [_ w586]
          tunnel: w536 -> [_ w585]
          tunnel: w535 -> [_ w584]
          tunnel: w534 -> [_ w583]
          tunnel: w533 -> [_ w581]
          tunnel: w532 -> [_ w580]
          tunnel: w531 -> [_ w579]
          tunnel: w530 -> [_ w578]
          tunnel: w529 -> [_ w577]
          tunnel: w528 -> [_ w576]
          frame False {
            w574 = 0.0
          }
          frame True {
            n286 = Subtract(x=w639, y=w638) -> (x-y=w768:dbl)
            n287 = Subtract(x=w636, y=w634) -> (x-y=w769:dbl)
            n288 = Multiply(x=w639, y=w640) -> (x*y=w652:dbl)
            n289 = Multiply(x=w638, y=w641) -> (x*y=w653:dbl)
            n290 = Multiply(x=w637, y=w635) -> (x*y=w654:dbl)
            n291 = Multiply(x=w636, y=w640) -> (x*y=w655:dbl)
            n292 = Multiply(x=w634, y=w641) -> (x*y=w656:dbl)
            n293 = Multiply(x=w633, y=w635) -> (x*y=w657:dbl)
            n294 = Subtract(x=w639, y=w637) -> (x-y=w758:dbl)
            n295 = Subtract(x=w636, y=w633) -> (x-y=w759:dbl)
            n296 = Subtract(x=w638, y=w637) -> (x-y=w767:dbl)
            n297 = Subtract(x=w634, y=w633) -> (x-y=w766:dbl)
            n298 = Index Array(array=w752, index=w712) -> (element=w751:dbl)
            n299 = Index Array(array=w725, index=w712) -> (element=w733:dbl)
            n300 = Index Array(array=w711, index=w712) -> (element=w718:dbl)
            n301 = Index Array(array=w742, index=w712) -> (element=w745:dbl)
            n302 = Index Array(array=w710, index=w712) -> (element=w723:dbl)
            n303 = Index Array(array=w724, index=w712) -> (element=w738:dbl)
            n304 = Compound Arithmetic op=ADD(w640, w641, w635) -> (w648:dbl)
            n305 = Compound Arithmetic op=ADD(w640, w641, w635) -> (w650:dbl)
            n306 = Compound Arithmetic op=ADD(w640, w641, w635) -> (w671:dbl)
            n307 = Compound Arithmetic op=ADD(w640, w641, w635) -> (w664:dbl)
            n308 = Number To Fractional String(number=w638) -> (F-format string=w700:string)  [unwired: 3 in]
            n309 = Number To Fractional String(number=w634) -> (F-format string=w697:string)  [unwired: 3 in]
            n310 = Number To Fractional String(number=w637) -> (F-format string=w695:string)  [unwired: 3 in]
            n311 = Number To Fractional String(number=w633) -> (F-format string=w692:string)  [unwired: 3 in]
            n312 = Number To Fractional String(number=w639) -> (F-format string=w705:string)  [unwired: 3 in]
            n313 = Number To Fractional String(number=w636) -> (F-format string=w702:string)  [unwired: 3 in]
            n314 = Subtract(x=w712, y=1) -> (x-y=w754:i32)
            n315 = Subtract(x=w712, y=1) -> (x-y=w731:i32)
            n316 = Subtract(x=w712, y=1) -> (x-y=w716:i32)
            n317 = Subtract(x=w712, y=1) -> (x-y=w743:i32)
            n318 = Subtract(x=w712, y=1) -> (x-y=w708:i32)
            n319 = Subtract(x=w712, y=1) -> (x-y=w726:i32)
            n320 = Square(x=w768) -> (x^2=w770:dbl)
            n321 = Square(x=w769) -> (x^2=w771:dbl)
            n322 = Square(x=w758) -> (x^2=w760:dbl)
            n323 = Square(x=w759) -> (x^2=w761:dbl)
            n324 = Square(x=w767) -> (x^2=w765:dbl)
            n325 = Square(x=w766) -> (x^2=w764:dbl)
            n326 = Index Array(array=w752, index=w754) -> (element=w750:dbl)
            n327 = Index Array(array=w725, index=w731) -> (element=w734:dbl)
            n328 = Index Array(array=w711, index=w716) -> (element=w719:dbl)
            n329 = Index Array(array=w742, index=w743) -> (element=w746:dbl)
            n330 = Index Array(array=w710, index=w708) -> (element=w722:dbl)
            n331 = Index Array(array=w724, index=w726) -> (element=w737:dbl)
            n332 = Compound Arithmetic op=ADD(w652, w653, w654) -> (w649:dbl)
            n333 = Compound Arithmetic op=ADD(w655, w656, w657) -> (w651:dbl)
            n334 = Add(x=w770, y=w771) -> (x+y=w772:dbl)
            n335 = Subtract(x=w751, y=w750) -> (x-y=w749:dbl)
            n336 = Subtract(x=w733, y=w734) -> (x-y=w735:dbl)
            n337 = Subtract(x=w718, y=w719) -> (x-y=w720:dbl)
            n338 = Subtract(x=w745, y=w746) -> (x-y=w747:dbl)
            n339 = Subtract(x=w723, y=w722) -> (x-y=w721:dbl)
            n340 = Subtract(x=w738, y=w737) -> (x-y=w736:dbl)
            n341 = Add(x=w760, y=w761) -> (x+y=w762:dbl)
            n342 = Add(x=w765, y=w764) -> (x+y=w763:dbl)
            n343 = Divide(x=w649, y=w648) -> (x/y=w590:dbl)
            n344 = Divide(x=w651, y=w650) -> (x/y=w589:dbl)
            n345 = Concatenate Strings("(" ("字符串"), w700, "," ("字符串"), w697, ")" ("字符串")) -> (→"p2 2":string)
            n346 = Reciprocal(x=w748) -> (1/x=w709:dbl)
            n347 = Concatenate Strings("(" ("字符串"), w695, "," ("字符串"), w692, ")" ("字符串")) -> (→"p3":string)
            n348 = Concatenate Strings("(" ("字符串"), w705, "," ("字符串"), w702, ")" ("字符串")) -> (→"p1":string)
            n349 = Multiply(x=w749, y=w709) -> (x*y=w605:dbl)
            n350 = Multiply(x=w735, y=w709) -> (x*y=w601:dbl)
            n351 = Multiply(x=w720, y=w709) -> (x*y=w597:dbl)
            n352 = Multiply(x=w747, y=w709) -> (x*y=w604:dbl)
            n353 = Multiply(x=w721, y=w709) -> (x*y=w595:dbl)
            n354 = Multiply(x=w736, y=w709) -> (x*y=w599:dbl)
            n355 = Square Root(x=w772) -> (sqrt(x)=w757:dbl)
            "d12" <- w757
            n356 = Number To Fractional String(number=w590) -> (F-format string=w645:string)  [unwired: 3 in]
            n357 = Number To Fractional String(number=w589) -> (F-format string=w646:string)  [unwired: 3 in]
            n358 = Square Root(x=w762) -> (sqrt(x)=w756:dbl)
            "d13" <- w756
            n359 = Square Root(x=w763) -> (sqrt(x)=w755:dbl)
            "d23" <- w755
            n360 = case shown="真" w607 {
              tunnel: w605 -> [w807 w822]
              tunnel: w604 -> [w806 w821]
              tunnel: [w807 w817] -> w603
              tunnel: [w806 w816] -> w602
              tunnel: w601 -> [w805 w815]
              tunnel: [w805 w814] -> w600
              tunnel: w599 -> [w804 w813]
              tunnel: [w804 w812] -> w598
              tunnel: w597 -> [w803 w811]
              tunnel: [w803 w810] -> w596
              tunnel: w595 -> [w802 w809]
              tunnel: [w802 w808] -> w594
              frame False {
              }
              frame True {
                n361 = call <vilib>:"1D Rectangular to Polar PtByPt.vi"("y"=w821, "x"=w822) -> ("phase"=w820:dbl, "magnitude"=w817:dbl)
                n362 = call <vilib>:"1D Rectangular to Polar PtByPt.vi"("y"=w809, "x"=w811) -> ("phase"=w818:dbl, "magnitude"=w810:dbl)
                n363 = call <vilib>:"1D Rectangular to Polar PtByPt.vi"("y"=w813, "x"=w815) -> ("phase"=w819:dbl, "magnitude"=w814:dbl)
                n364 = expression code="(x/pi)*180.0" "x"(w820) -> (w816:dbl)
                n365 = expression code="(x/pi)*180.0" "x"(w818) -> (w808:dbl)
                n366 = expression code="(x/pi)*180.0" "x"(w819) -> (w812:dbl)
              }
            }
            n367 = Multiply(x=w605, y=w640) -> (x*y=w676:dbl)
            n368 = Multiply(x=w601, y=w641) -> (x*y=w674:dbl)
            n369 = Multiply(x=w597, y=w635) -> (x*y=w673:dbl)
            n370 = Multiply(x=w604, y=w640) -> (x*y=w675:dbl)
            n371 = Multiply(x=w595, y=w635) -> (x*y=w662:dbl)
            n372 = Multiply(x=w599, y=w641) -> (x*y=w661:dbl)
            n373 = Square(x=w604) -> (x^2=w741:dbl)
            n374 = Square(x=w605) -> (x^2=w740:dbl)
            n375 = Square(x=w601) -> (x^2=w730:dbl)
            n376 = Square(x=w599) -> (x^2=w729:dbl)
            n377 = Square(x=w597) -> (x^2=w715:dbl)
            n378 = Square(x=w595) -> (x^2=w714:dbl)
            n379 = Add(x=w741, y=w740) -> (x+y=w739:dbl)
            n380 = Add(x=w730, y=w729) -> (x+y=w728:dbl)
            n381 = Add(x=w715, y=w714) -> (x+y=w713:dbl)
            n382 = Compound Arithmetic op=ADD(w676, w674, w673) -> (w672:dbl)
            n383 = Compound Arithmetic op=ADD(w675, w662, w661) -> (w663:dbl)
            n384 = Concatenate Strings("(" ("字符串"), w645, "," ("字符串"), w646, ")" ("字符串")) -> (→"pmc":string)
            n385 = Divide(x=w672, y=w671) -> (x/y=w622:dbl)
            n386 = Divide(x=w663, y=w664) -> (x/y=w623:dbl)
            n387 = Square Root(x=w739) -> (sqrt(x)=w610:dbl)
            "s1" <- w610
            n388 = Square Root(x=w728) -> (sqrt(x)=w608:dbl)
            "s2" <- w608
            n389 = Square Root(x=w713) -> (sqrt(x)=w609:dbl)
            "s3" <- w609
            n390 = Square(x=w622) -> (x^2=w660:dbl)
            n391 = Square(x=w623) -> (x^2=w659:dbl)
            n392 = Number To Fractional String(number=w622) -> (F-format string=w669:string)  [unwired: 3 in]
            n393 = Number To Fractional String(number=w623) -> (F-format string=w666:string)  [unwired: 3 in]
            n394 = Add(x=w660, y=w659) -> (x+y=w658:dbl)
            n395 = Number To Fractional String(number=w603) -> (F-format string=w688:string)  [unwired: 3 in]
            n396 = Number To Fractional String(number=w602) -> (F-format string=w691:string)  [unwired: 3 in]
            n397 = Number To Fractional String(number=w596) -> (F-format string=w678:string)  [unwired: 3 in]
            n398 = Number To Fractional String(number=w594) -> (F-format string=w681:string)  [unwired: 3 in]
            n399 = Number To Fractional String(number=w600) -> (F-format string=w683:string)  [unwired: 3 in]
            n400 = Number To Fractional String(number=w598) -> (F-format string=w686:string)  [unwired: 3 in]
            n401 = Square Root(x=w658) -> (sqrt(x)=w624:dbl)
            "smc" <- w624
            n402 = Concatenate Strings("(" ("字符串"), w669, "," ("字符串"), w666, ")" ("字符串")) -> (→"vmc":string)
            n403 = Concatenate Strings("(" ("字符串"), w688, "," ("字符串"), w691, ")" ("字符串")) -> (→"v1":string)
            n404 = Concatenate Strings("(" ("字符串"), w678, "," ("字符串"), w681, ")" ("字符串")) -> (→"v3":string)
            n405 = Concatenate Strings("(" ("字符串"), w683, "," ("字符串"), w686, ")" ("字符串")) -> (→"v2":string)
            n406 = Divide(x=w622, y=w624) -> (x/y=w621:dbl)
            n407 = Divide(x=w623, y=w624) -> (x/y=w619:dbl)
            n408 = Divide(x=w620, y=40.0) -> (x/y=w611:dbl)
            n409 = Multiply(x=w621, y=w611) -> (x*y=w618:dbl)
            n410 = Multiply(x=w619, y=w611) -> (x*y=w617:dbl)
            n411 = Add(x=w618, y=w590) -> (x+y=w615:dbl)
            n412 = Add(x=w589, y=w617) -> (x+y=w616:dbl)
            n413 = Build Array(w590) -> (w627:dbl[])
            n414 = Build Array(w589) -> (w591:dbl[])
            n415 = Build Array(w615) -> (w614:dbl[])
            n416 = Build Array(w616) -> (w613:dbl[])
            n417 = Bundle(w627, w591) -> (w626:cluster{dbl[], dbl[]})  [unwired: 1 out]
            n418 = Bundle(w614, w613) -> (w592:cluster{dbl[], dbl[]})  [unwired: 1 out]
            n419 = case shown="真" "显示物体半径？" {
              tunnel: w626 -> [w774 w801]
              tunnel: [w776 w800] -> w625
              tunnel: w593 -> [w775 w799]
              tunnel: w592 -> [w773 w798]
              tunnel: w588 -> [_ w795]
              tunnel: w587 -> [_ w794]
              tunnel: w586 -> [_ w789]
              tunnel: w585 -> [_ w788]
              tunnel: w584 -> [_ w787]
              tunnel: w583 -> [_ w786]
              tunnel: w581 -> [_ w782]
              tunnel: w580 -> [_ w781]
              tunnel: w579 -> [_ w780]
              tunnel: w578 -> [_ w779]
              tunnel: w577 -> [_ w778]
              tunnel: w576 -> [_ w777]
              frame False {
                n420 = Build Array (concatenate)(w775, w774, w773) -> (w776:cluster{"Y-out":dbl[], "Y-out":dbl[]}[])
              }
              frame True {
                n421 = Add(x=w782, y=w794) -> (x+y=w797:dbl[])
                n422 = Add(x=w781, y=w795) -> (x+y=w796:dbl[])
                n423 = Add(x=w780, y=w789) -> (x+y=w793:dbl[])
                n424 = Add(x=w779, y=w788) -> (x+y=w792:dbl[])
                n425 = Add(x=w778, y=w787) -> (x+y=w791:dbl[])
                n426 = Add(x=w777, y=w786) -> (x+y=w790:dbl[])
                n427 = Bundle(w797, w796) -> (w785:cluster{dbl[], dbl[]})  [unwired: 1 in]
                n428 = Bundle(w793, w792) -> (w784:cluster{dbl[], dbl[]})  [unwired: 1 in]
                n429 = Bundle(w791, w790) -> (w783:cluster{dbl[], dbl[]})  [unwired: 1 in]
                n430 = Build Array (concatenate)(w799, w801, w798, w785, w784, w783) -> (w800:cluster{"Y-out":dbl[], "Y-out":dbl[]}[])
              }
            }
          }
        }
        "?" <- w541
        "t" <- w560
      }
      n431 = Divide(x=w141, y=2.0) -> (x/y=w135:dbl)
      n432 = Divide(x=w145, y=2.0) -> (x/y=w131:dbl)
      n433 = Divide(x=w137, y=2.0) -> (x/y=w132:dbl)
      n434 = Add(x=w135, y=w131) -> (x+y=w136:dbl)
      n435 = Subtract(x=w135, y=w131) -> (x-y=w134:dbl)
      n436 = Add(x=w132, y=w131) -> (x+y=w133:dbl)
      n437 = Subtract(x=w132, y=w131) -> (x-y=w130:dbl)
      n438 = Divide(x=w145, y=40.0) -> (x/y=w223:dbl)
      n439 = case shown="真" "自动缩放？" {
        tunnel: w223 -> [_ w520]
        tunnel: w136 -> [_ w521]
        tunnel: w134 -> [_ w526]
        tunnel: w133 -> [_ w523]
        tunnel: w130 -> [_ w525]
        frame False {
        }
        frame True {
          n440 = Add(x=w521, y=w520) -> (x+y=w519:dbl)
          n441 = Subtract(x=w526, y=w520) -> (x-y=w527:dbl)
          n442 = Add(x=w523, y=w520) -> (x+y=w522:dbl)
          n443 = Subtract(x=w525, y=w520) -> (x-y=w524:dbl)
          n444 = property class="XYGraph (严格)"("XScale.Maximum"=w519) -> ()  [unwired: 2 in, 2 out]
          n445 = property class="XYGraph (严格)"("XScale.Minimum"=w527) -> ()  [unwired: 2 in, 2 out]
          n446 = property class="XYGraph (严格)"("YScale.Maximum"=w522) -> ()  [unwired: 2 in, 2 out]
          n447 = property class="XYGraph (严格)"("YScale.Minimum"=w524) -> ()  [unwired: 2 in, 2 out]
        }
      }
      n448 = Array Max & Min(array=w241) -> (max value=→"dmax12":dbl, max index (indices)=w238:i32, min value=→"dmin12":dbl, min index (indices)=w237:i32)
      n449 = Array Max & Min(array=w236) -> (max value=→"dmax13":dbl, max index (indices)=w233:i32, min value=→"dmin13":dbl, min index (indices)=w232:i32)
      n450 = Array Max & Min(array=w231) -> (max value=→"dmax23":dbl, max index (indices)=w228:i32, min value=→"dmin23":dbl, min index (indices)=w227:i32)
      n451 = Delete From Array(array=w198, length=1 ("长度"), index=0 ("索引")) -> (array with subset deleted=w197:dbl[])  [unwired: 1 out]
      n452 = Delete From Array(array=w194, length=1 ("长度"), index=0 ("索引")) -> (array with subset deleted=w193:dbl[])  [unwired: 1 out]
      n453 = Delete From Array(array=w190, length=1 ("长度"), index=0 ("索引")) -> (array with subset deleted=w189:dbl[])  [unwired: 1 out]
      n454 = Array Max & Min(array=w197) -> (max value=→"smax1":dbl, max index (indices)=w212:i32, min value=→"smin1":dbl, min index (indices)=w211:i32)
      n455 = Array Max & Min(array=w193) -> (max value=→"smax2":dbl, max index (indices)=w209:i32, min value=→"smin2":dbl, min index (indices)=w207:i32)
      n456 = Array Max & Min(array=w189) -> (max value=→"smax3":dbl, max index (indices)=w205:i32, min value=→"smin3":dbl, min index (indices)=w203:i32)
      n457 = Divide(x=w238, y=w202) -> (x/y=→"tdmax12":dbl)
      n458 = Divide(x=w237, y=w202) -> (x/y=→"tdmin12":dbl)
      n459 = Divide(x=w233, y=w202) -> (x/y=→"tdmax23":dbl)
      n460 = Divide(x=w227, y=w202) -> (x/y=→"tdmin13":dbl)
      n461 = Divide(x=w232, y=w202) -> (x/y=→"tdmin23":dbl)
      n462 = Divide(x=w228, y=w202) -> (x/y=→"tdmax13":dbl)
      n463 = Divide(x=w212, y=w202) -> (x/y=→"tsmax1":dbl)
      n464 = Divide(x=w211, y=w202) -> (x/y=→"tsmin1":dbl)
      n465 = Divide(x=w209, y=w202) -> (x/y=→"tsmax2":dbl)
      n466 = Divide(x=w207, y=w202) -> (x/y=→"tsmin2":dbl)
      n467 = Divide(x=w205, y=w202) -> (x/y=→"tsmax3":dbl)
      n468 = Divide(x=w203, y=w202) -> (x/y=→"tsmin3":dbl)
    }
  }
